vi "Test Empty Path.vi"(11 "Test Case In":refnum<class "Test File Exists.lvclass">) -> (0 "error out":errorcluster, 3 "Test Case Out":refnum<class "Test File Exists.lvclass">)   [LabVIEW 2024, in "Test File Exists.lvclass"]
uses:
  Test File Exists.lvclass
  C:/Program Files/National Instruments/LabVIEW 2025/vi.lib/Astemes/LUnit/Test Case.lvclass
  <vilib>/Astemes/LUnit/Test Case.lvclass/Test Case.ctl
  <vilib>/Astemes/LUnit/Append Pass Result.vi
  <vilib>/Astemes/LUnit/Append Fail Result.vi
  <vilib>/Astemes/LUnit/Run In UI.vi
  <vilib>/Utility/error.llb/Clear Errors.vi
  Source/Common Helpers.lvlib
  <vilib>/Astemes/LUnit/Test Case.lvclass
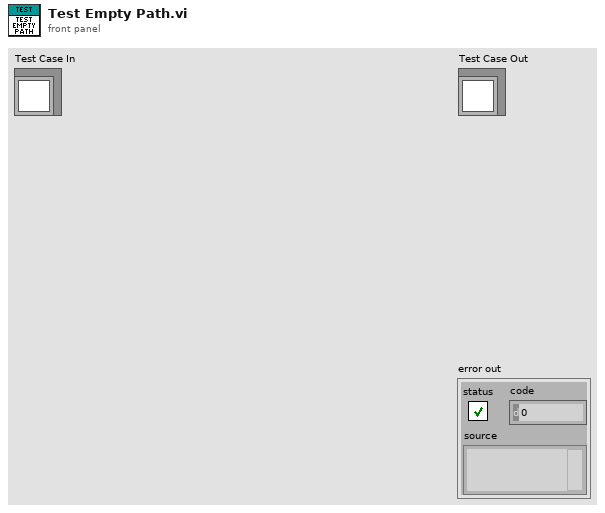
[diagram p1: front panel]
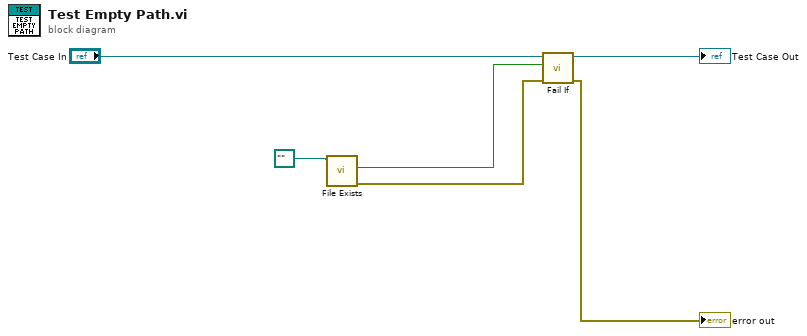
[diagram p0: block diagram]
diagram:
  n1 = call "File Exists.vi"("File Path"=path "") -> ("error out"=w1:errorcluster, "Exists"=w2:bool)  [unwired: 8 in, 1 out]
  n2 = call <vilib>:"Fail If.vi"("error in (no error)"=w1, "Fail?"=w2, "LUnit Test Case In"="Test Case In") -> ("error out"=→"error out":errorcluster, "LUnit Test Case Out"=→"Test Case Out":refnum<class "Test File Exists.lvclass">)  [unwired: 7 in]
